vi "StimError.vi"(0 "VISA Resource Name":refnum<visa-resource-name>="COM1", 5 "Enable":bool=TRUE, 11 "error in (no error)":errorcluster) -> (3 "Hasomed Status":string, 4 "VISA resource name out":refnum<visa-resource-name>, 6 "No Error":bool=TRUE, 15 "error out":errorcluster)   [LabVIEW 2017]
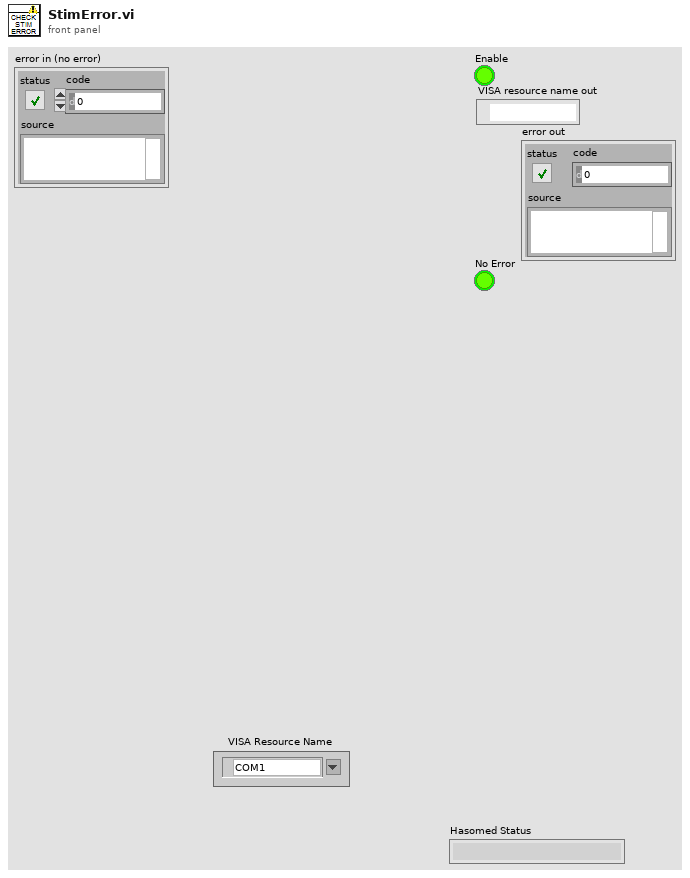
[diagram p1: front panel]
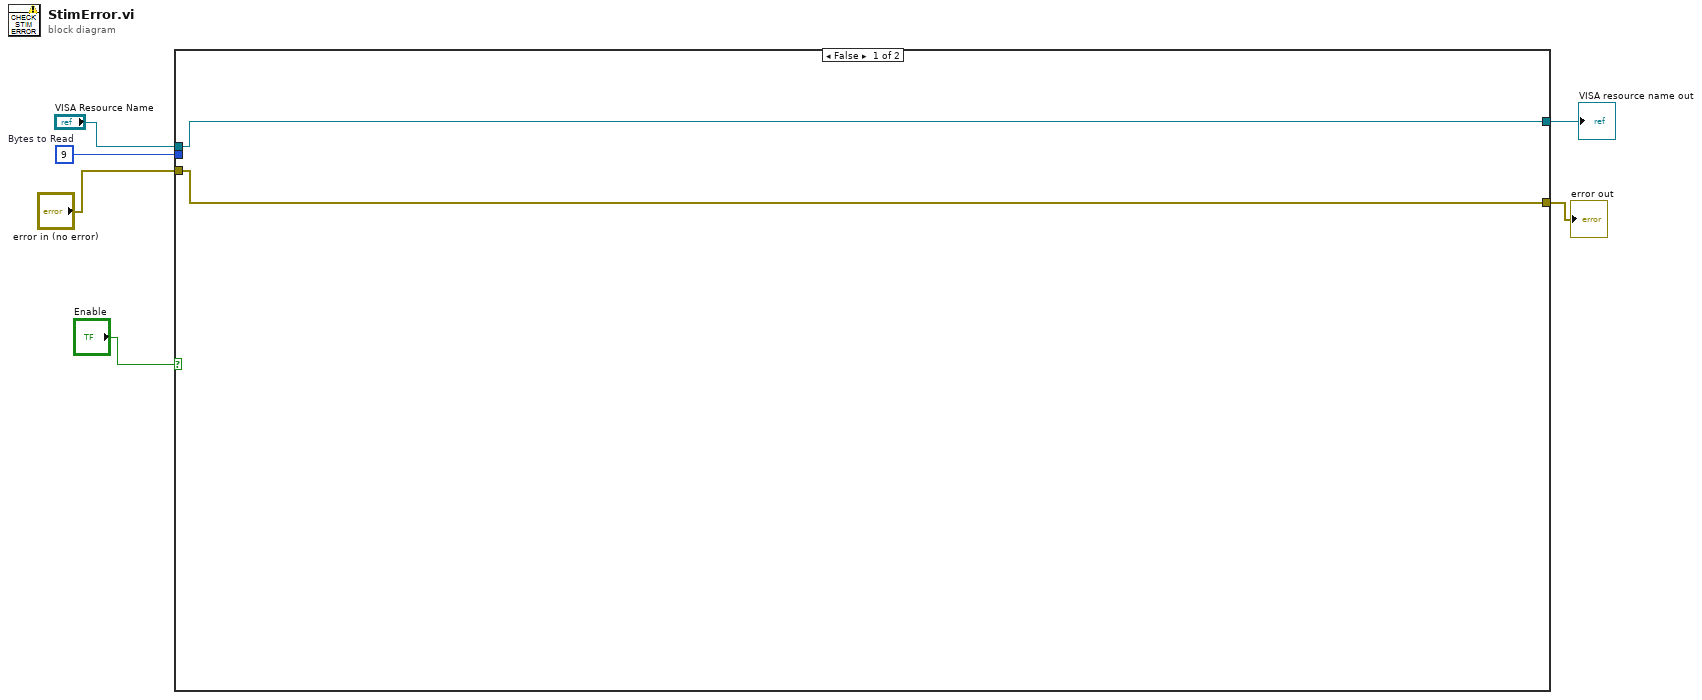
[diagram p0: block diagram]
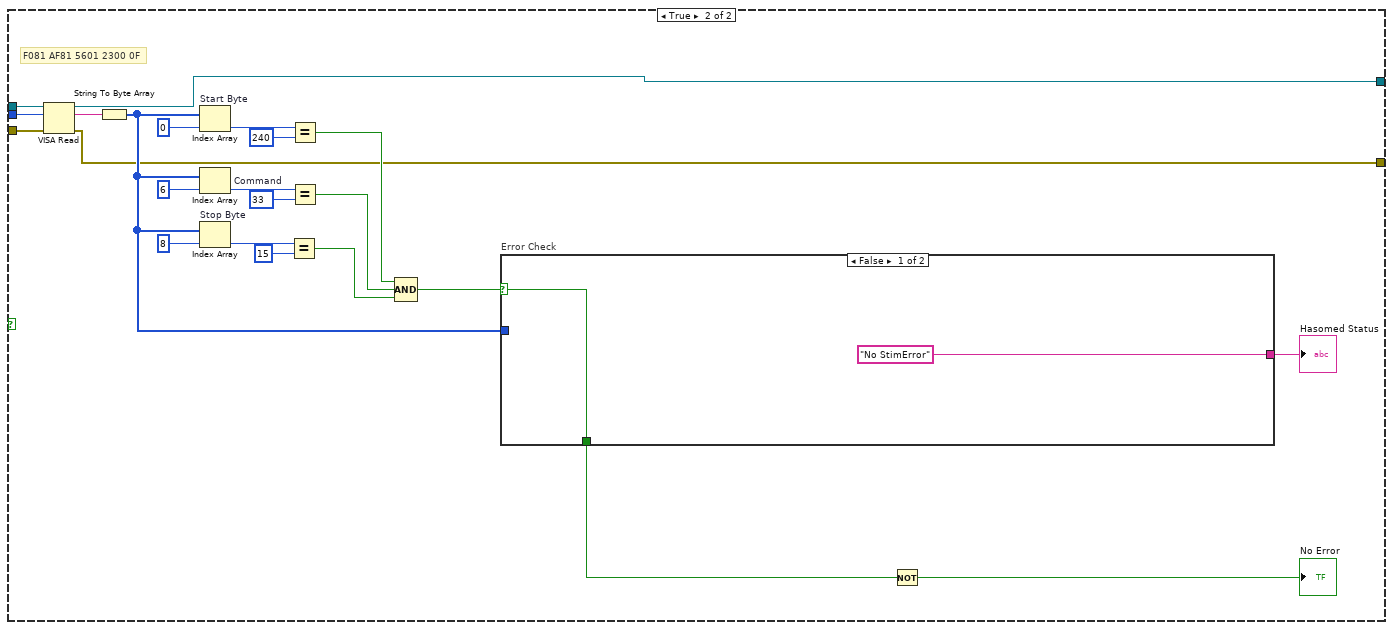
[diagram p2: hidden frame]
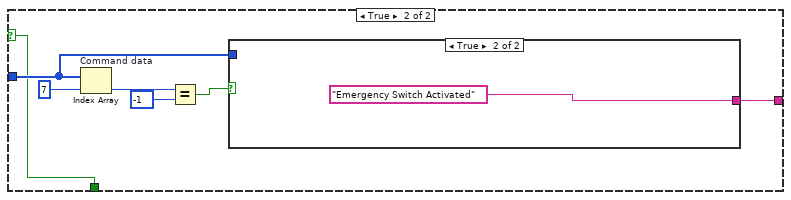
[diagram p3: hidden frame]
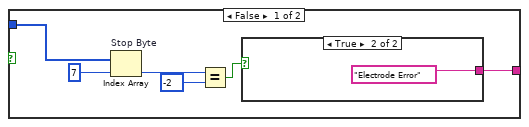
[diagram p4: hidden frame]
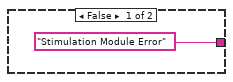
[diagram p5: hidden frame]
diagram:
  w6 = 9  # Bytes to Read
  n1 = case shown="False" "Enable" {
    tunnel: w6 -> [_ w24]
    tunnel: "VISA Resource Name" -> [w8 w15]
    tunnel: "error in (no error)" -> [w7 w11]
    tunnel: [w7 w10] -> w2
    tunnel: [w8 w9] -> w1
    frame False {
    }
    frame True {
      # "F081 AF81 5601 2300 0F"
      n2 = VISA Read(VISA resource name=w15, byte count=w24, error in (no error)=w11) -> (VISA resource name out=w9:refnum<visa-resource-name>, read buffer=w18:string, error out=w10:errorcluster)  [unwired: 1 out]
      n3 = String To Byte Array(string=w18) -> (unsigned byte array=w16:u8[])
      n4 = Index Array "Start Byte"(array=w16, index=0) -> (element=w27:u8)
      n5 = Index Array "Command"(array=w16, index=6) -> (element=w25:u8)
      n6 = Index Array "Stop Byte"(array=w16, index=8) -> (element=w21:u8)
      n7 = Equal?(x=w21, y=u16 15) -> (x = y?=w17:bool)
      n8 = Equal?(x=w27, y=u16 240) -> (x = y?=w19:bool)
      n9 = Equal?(x=w25, y=u16 33) -> (x = y?=w20:bool)
      n10 = Compound Arithmetic op=AND(w19, w20, w17) -> (w14:bool)
      n11 = case "Error Check" shown="False" w14 {
        selector: w14 -> [w32 w34]
        tunnel: ["No StimError" w40] -> w31
        tunnel: w16 -> [_ w35]
        tunnel: [w32 w34] -> w12
        frame False {
        }
        frame True {
          n12 = Index Array "Command data"(array=w35, index=7) -> (element=w39:u8)
          n13 = Equal?(x=w39, y=i8 -1) -> (x = y?=w36:bool)
          n14 = case shown="True" w36 {
            tunnel: [w41 "Emergency Switch Activated"] -> w40
            tunnel: w35 -> [w43 _]
            frame False {
              n15 = Index Array "Stop Byte"(array=w43, index=7) -> (element=w46:u8)
              n16 = Equal?(x=w46, y=i8 -2) -> (x = y?=w42:bool)
              n17 = case shown="True" w42 {
                tunnel: ["Stimulation Module Error" "Electrode Error"] -> w41
                frame False {
                }
                frame True {
                }
              }
            }
            frame True {
            }
          }
        }
      }
      "Hasomed Status" <- w31
      n18 = Not(x=w12) -> (.not. x?=→"No Error":bool)
    }
  }
  "error out" <- w2
  "VISA resource name out" <- w1
